vi "Capture@ROISave__Parameter.vi"(1 "ParamterIn":string) -> (0 "ParamterOut":string)   [LabVIEW 2020]
uses:
  MainFrame/Global.vi
panel:
  out "Image":T1(plugin-control)
  in  "Picture":string(combo)
  in  "CamName":string(combo)
  in  "Confirm":bool
  # "Capture@ROISave $Capture,$Picture"
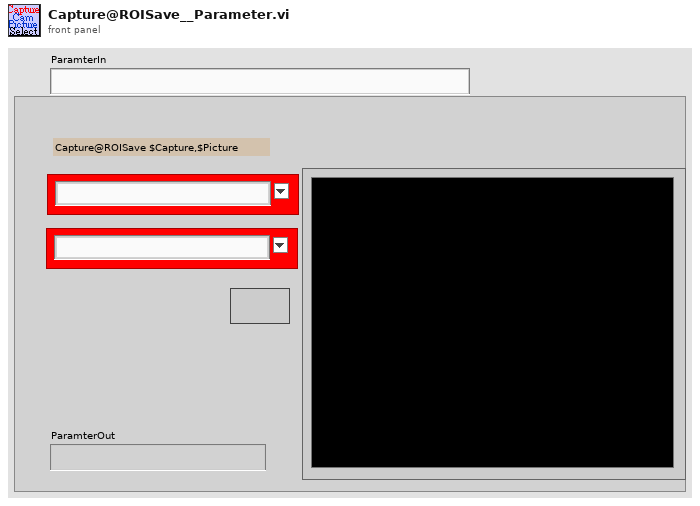
[diagram p1: front panel]
types:
  T1 = typedef "IMAQ Image.ctl" = refnum<image>
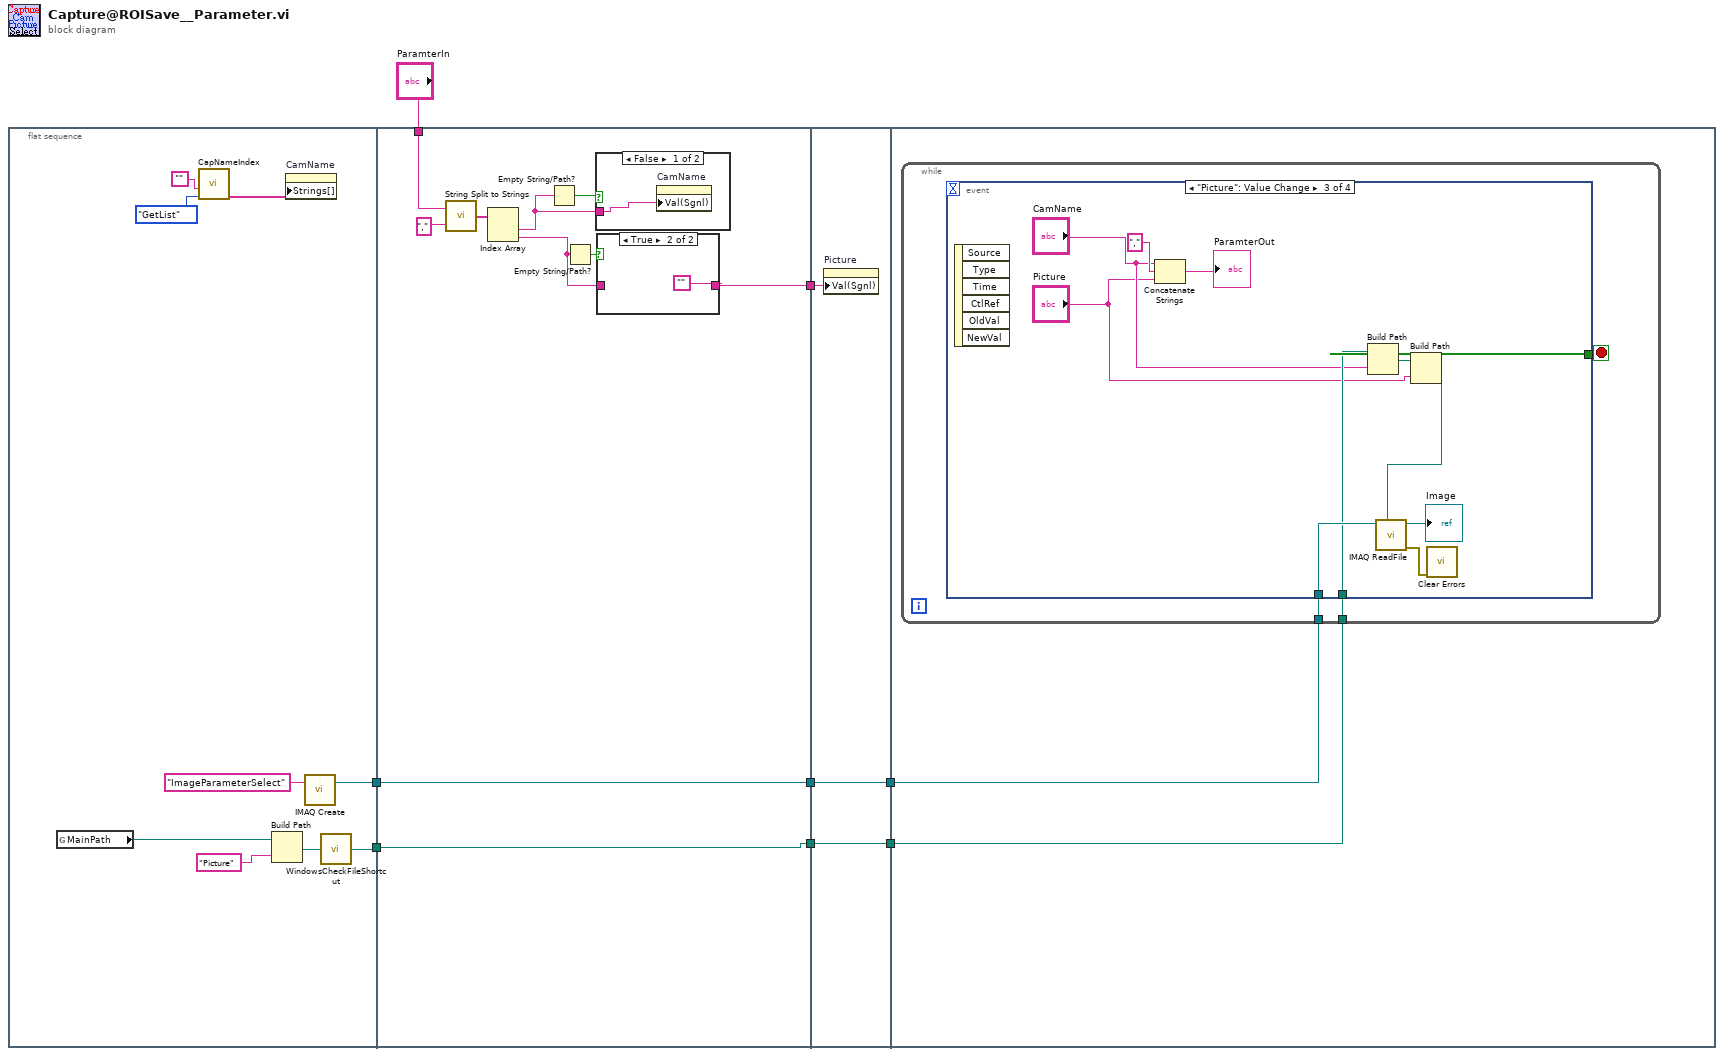
[diagram p0: block diagram]
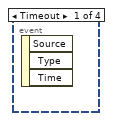
[diagram p4: hidden frame]
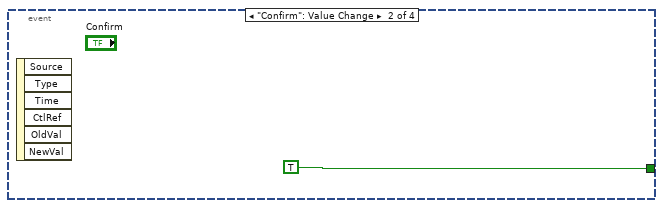
[diagram p5: hidden frame]
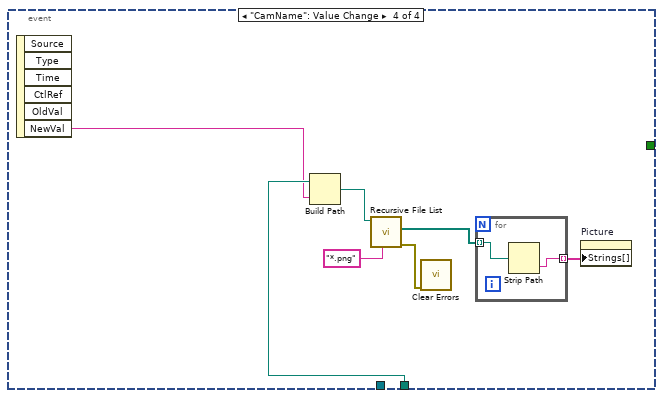
[diagram p6: hidden frame]
diagram:
  n1 = flat-sequence {
    tunnel: [w13] -> w7
    tunnel: [w9] -> w2
    tunnel: "ParamterIn" -> [w25]
    tunnel: w7 -> [w21]
    tunnel: [w21] -> w6
    tunnel: [w19] -> w3
    tunnel: w2 -> [w19]
    tunnel: [w18] -> w1
    tunnel: w6 -> [w33]
    tunnel: [w33] -> w5
    tunnel: [w32] -> w4
    tunnel: w3 -> [w32]
    tunnel: w1 -> [w31]
    tunnel: w5 -> [w35]
    tunnel: w4 -> [w34]
    frame #0 {
      n2 = global read "Global.vi" "MainPath"() -> (w11:path)
      n3 = call "CapNameIndex.vi"("OP"=enum16{"AddCam", "GetIndex", "Init", "GetList"}."GetList", "CamName"="") -> ("DeviceList"=w16:string[])  [unwired: 2 in, 3 out]
      n4 = Build Path(base path=w11, name or relative path="Picture") -> (appended path=w10:path)
      n5 = property on="CamName" class="CmbBox"("Strings[]"=w16) -> ()  [unwired: 2 in, 2 out]
      n6 = call "IMAQ Create"("Image Name"="ImageParameterSelect") -> ("New Image"=w13:T1)  [unwired: 4 in, 1 out]
      n7 = call "WindowsCheckFileShortcut.vi"("LinkPath"=w10) -> ("TargetPath"=w9:path)  [unwired: 4 in]
    }
    frame #1 {
      n8 = call "String Split to Strings.vi"("search string/char (-)"=",", "String"=w25) -> ("Array"=w27:string[])
      n9 = Index Array(array=w27) -> (element #1=w20:string, element #2=w22:string)  [unwired: 2 in]
      n10 = Empty String/Path?(string/path=w20) -> (empty?=w24:bool)
      n11 = Empty String/Path?(string/path=w22) -> (empty?=w23:bool)
      n12 = case shown="False" w24 {
        tunnel: w20 -> [w30 _]
        frame False {
          n13 = property on="CamName" class="CmbBox"("Val(Sgnl)"=w30) -> ()  [unwired: 2 in, 2 out]
        }
        frame True {
        }
      }
      n14 = case shown="True" w23 {
        tunnel: [w28 ""] -> w18
        tunnel: w22 -> [w28 _]
        frame False {
        }
        frame True {
        }
      }
    }
    frame #2 {
      n15 = property on="Picture" class="CmbBox"("Val(Sgnl)"=w31) -> ()  [unwired: 2 in, 2 out]
    }
    frame #3 {
      n16 = while {
        tunnel: w35 -> [w37]
        tunnel: w34 -> [w36]
        stop <- w38 stop-if-true
        n17 = event shown="[2] \"Picture\": Value Change" {
          selector: _ -> [_ _ _ _]
          dyn-events: _ -> [_ _ _ _]
          timeout: _ -> [_ _ _ _]
          tunnel: [_ TRUE _ _] -> w38
          tunnel: w37 -> [_ _ w47 _]
          tunnel: w36 -> [_ _ w46 w53]
          event Timeout {
            n18 = event-data() -> ()  [unwired: 1 in, 3 out]
          }
          event "Confirm": Value Change {
            n19 = event-data() -> ()  [unwired: 1 in, 6 out]
          }
          event "Picture": Value Change {
            n20 = event-data() -> ()  [unwired: 1 in, 6 out]
            n21 = Concatenate Strings("CamName", "," ("string"), "Picture") -> (→"ParamterOut":string)
            n22 = Build Path(base path=w46, name or relative path="CamName") -> (appended path=w44:path)
            n23 = Build Path(base path=w44, name or relative path="Picture") -> (appended path=w42:path)
            n24 = call "IMAQ ReadFile"("File Path"=w42, "Image"=w47) -> ("error out"=w41:errorcluster, "Image Out"=→"Image":T1)  [unwired: 5 in, 3 out]
            n25 = call <vilib>:"Clear Errors.vi"("error in (no error)"=w41) -> ()  [unwired: 5 in, 2 out]
          }
          event "CamName": Value Change {
            n26 = event-data() -> ("NewVal"=w52:string)  [unwired: 1 in, 5 out]
            n27 = Build Path(base path=w53, name or relative path=w52) -> (appended path=w51:path)
            n28 = call <vilib>:"Recursive File List.vi"("pattern"="*.png", "Folder Path"=w51) -> ("error out"=w50:errorcluster, "All Files in Dir"=w55:path[])  [unwired: 5 in, 3 out]
            n29 = call <vilib>:"Clear Errors.vi"("error in (no error)"=w50) -> ()  [unwired: 5 in, 2 out]
            n30 = for {
              tunnel: w55 -> [w58] mode=indexing
              tunnel: [w57] -> w56 mode=indexing
              n31 = Strip Path(path=w58) -> (name=w57:string)  [unwired: 1 out]
            }
            n32 = property on="Picture" class="CmbBox"("Strings[]"=w56) -> ()  [unwired: 2 in, 2 out]
          }
        }
      }
    }
  }
